vi "XY Graph to Igor Graph.vi"(8 "error in (no error)":errorcluster, 10 "XY Graph Reference":refnum<vi>, 11 "Path":path=path "C:/temp") -> (0 "error out":errorcluster, 3 "file":path=path "C:/Users/voodoo.SEAGATE/Desktop/datatest/datatest.000019.itx")   [LabVIEW 2020, in "Data.ITX.lvclass"]
uses:
  Data.ITX.lvclass
  graph_utilities/src/graph_utilities.lvclass
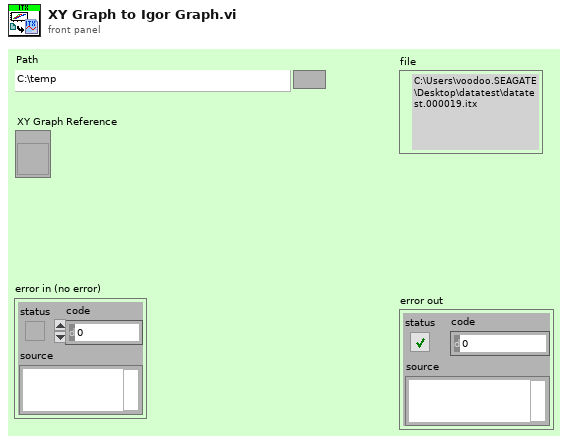
[diagram p1: front panel]
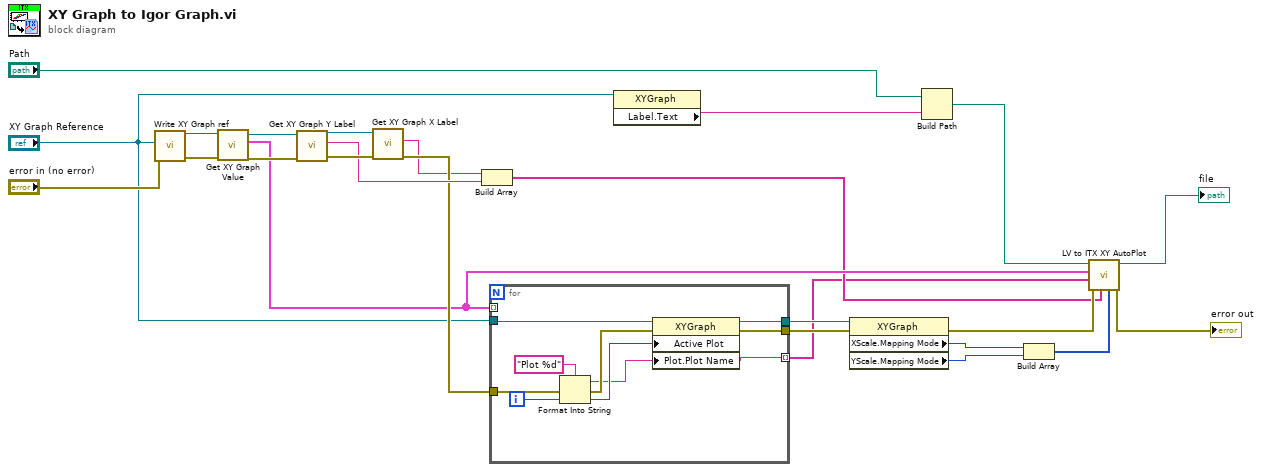
[diagram p0: block diagram]
diagram:
  n1 = call "Write XY Graph ref.vi"("error in (no error)"="error in (no error)", "XY Graph"="XY Graph Reference") -> ("error out"=w22:errorcluster, "graph_utilities out"=w23:refnum<class "graph_utilities.lvclass">)  [unwired: 8 in]
  n2 = call "Get XY Graph Value.vi"("error in (no error)"=w22, "graph_utilities in"=w23) -> ("error out"=w20:errorcluster, "Value"=w11:cluster{"X":dbl[], "Y":dbl[]}[], "graph_utilities out"=w21:refnum<class "graph_utilities.lvclass">)  [unwired: 7 in]
  n3 = call "Get XY Graph Y Label.vi"("error in (no error)"=w20, "graph_utilities in"=w21) -> ("error out"=w18:errorcluster, "Y Label"=w17:string, "graph_utilities out"=w19:refnum<class "graph_utilities.lvclass">)  [unwired: 7 in]
  n4 = call "Get XY Graph X Label.vi"("error in (no error)"=w18, "graph_utilities in"=w19) -> ("error out"=w15:errorcluster, "X Label"=w10:string)  [unwired: 7 in, 1 out]
  n5 = Build Array(w10, w17) -> (w9:string[])
  n6 = for {
    tunnel: "XY Graph Reference" -> [w33]
    tunnel: [w32] -> w16
    tunnel: w11 -> [_] mode=indexing
    tunnel: w15 -> [w29]
    tunnel: [w27] -> w14
    tunnel: [w26] -> w5 mode=indexing
    i -> [w30]
    n7 = Format Into String(format string="Plot %d", error in=w29, w30) -> (resulting string=w26:string, error out=w28:errorcluster)  [unwired: 1 in]
    n8 = property on="Property Node" class="XYGraph"(reference=w33, error in=w28, "Active Plot"=w30, "Plot.Plot Name"=w26) -> (reference out=w32:refnum<vi>, error out=w27:errorcluster)
  }
  n9 = property on="Property Node" class="XYGraph"(reference="XY Graph Reference") -> ("Label.Text"=w3:string)  [unwired: 1 in, 2 out]
  n10 = property on="Property Node" class="XYGraph"(reference=w16, error in=w14) -> (error out=w13:errorcluster, "XScale.Mapping Mode"=w25:u8, "YScale.Mapping Mode"=w24:u8)  [unwired: 1 out]
  n11 = Build Path(base path="Path", name or relative path=w3) -> (appended path=w1:path)
  n12 = Build Array(w25, w24) -> (w8:u8[])
  n13 = call "LV to ITX XY AutoPlot.vi"("X,Y Log"=w8, "X,Y Labels"=w9, "error in"=w13, "Plot Names"=w5, "XY-Data []"=w11, "path"=w1) -> ("error out"=→"error out":errorcluster, "file"=→"file":path)  [unwired: 4 in]
